vi "AddCommentToLog.vi"(8 "error in":errorcluster, 10 "Comment":string="Add comment to log...", 11 "UdsHandleIn":T1) -> (0 "error out":errorcluster, 3 "UdsHandleOut":T1)   [LabVIEW 2011, in "Konvolucio MUDS150628.lvlib"]
uses:
  <instrlib>/Konvolucio MUDS150628/Konvolucio MUDS150628.lvlib
  <instrlib>/Konvolucio MUDS150628/Types/UdsHandleType.ctl
  <instrlib>/Konvolucio MCAN120803/Types/MCanHandleType.ctl
  C:/Program Files/National Instruments/LabVIEW 2011/instr.lib/Konvolucio MCAN120803/Private/Konvolucio.MCAN120803.dll
  Konvolucio MCAN120803/Private/Konvolucio.MCAN120803.dll
  <instrlib>/Konvolucio MUDS150628/Private/UdsLogEvent.vi
  <instrlib>/Konvolucio MCAN120803/Konvolucio MCAN120803.lvlib
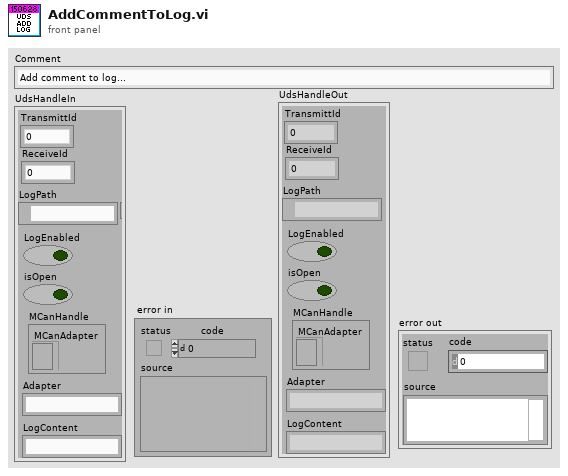
[diagram p1: front panel]
types:
  T1 = typedef "Konvolucio MUDS150628.lvlib/UdsHandleType.ctl" = cluster{"LogPath":path, "LogEnabled":bool, "isOpen":bool, "LogContent":string, "Adapter":string, "MCanHandle":T2, "TransmittId":u32, "ReceiveId":u32}
  T2 = typedef "Konvolucio MCAN120803.lvlib/MCanHandleType.ctl" = cluster{"MCanAdapter":refnum<k24>}
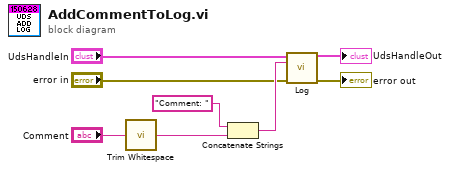
[diagram p0: block diagram]
diagram:
  n1 = call <vilib>:"Trim Whitespace.vi"("string"="Comment") -> ("trimmed string"=w6:string)  [unwired: 1 in]
  n2 = Concatenate Strings("Comment: " ("Msg"), w6) -> (w4:string)
  n3 = call-poly <instrlib>:"Log.vi"("UdsHandleIn"="UdsHandleIn", "EventMsg"=w4, "error in"="error in") -> ("UdsHandleOut"=→"UdsHandleOut":T1, "error out"=→"error out":errorcluster)  [unwired: 11 in]
